vi "Get Refnum Type Enum from TD.vi"(4 "Type Descriptor":refnum<class "TD.lvclass">) -> (1 "Refnum Subtype Enum":T1 format="%.0x")   [LabVIEW 2020]
doc: "Gets a Refnum Subtype Enumeration from a Type Descriptor Array."
uses:
  Refnum Subtype Enum.ctl
  661ef7ab-f49d-4acd-8334-4638e1c8a424.vi
  openg_variant.lvlib
  TD.lvclass
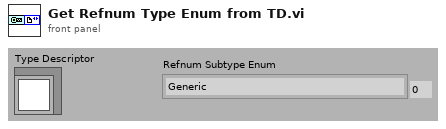
[diagram p1: front panel]
types:
  T1 = typedef "openg_variant.lvlib/Refnum Subtype Enum.ctl" = enum8{"Generic", "Datalog File Refnum", "Byte Stream File Refnum", "Device Refnum", "Occurence Refnum", "TCP Connection Refnum", "VISA Refnum (Obsolete)", "Automation Renum", "VI Server Refnum", "Menu Refnum", "IVI Refnum (Obsolete)", "IMAQ Session", "0x0C", "Datasocket Refnum", "VISA Resource", "IVI Logical Name", "UDP Connection Refnum", "Notifier Refnum", "Queue Refnum", "IrDA Refnum", "Hardware Plugin Refnum", "Hardware Plugin Tag Refnum", "DAQmx Refnum", "Event Registration Refnum", ".NET Refnum", "User Event Refnum", "0x1A", "Event Callback", "0x1C", "0x1D", "LabVIEW Class Instance", "Bluetooth", "Data Value References", "RT FIFO", "TDM Streaming"}
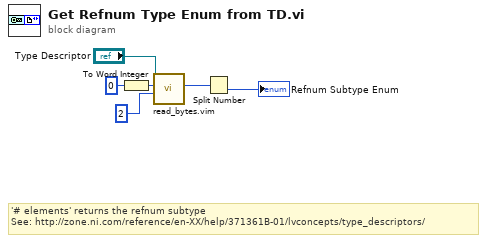
[diagram p0: block diagram]
diagram:
  # "'# elements' returns the refnum subtype\nSee: http://zone.ni.com/reference/en-XX/help/371361B-01/lvconcepts/type_descriptors/"
  n1 = To Word Integer(number=u8 0 ("data type")) -> (16bit integer=w4:i16)
  n2 = call "read_bytes.vim"("byte offset"=2, "data type"=w4, "Bytes in"="Type Descriptor") -> ("value"=w1:i16)  [unwired: 7 in, 1 out]
  n3 = Split Number(x=w1) -> (lo(x)=→"Refnum Subtype Enum":u8)  [unwired: 1 out]
